vi "CLK6.vi"(11 "Queue Out":T1) -> (0 "error out":errorcluster)   [LabVIEW 2015]
uses:
  Class/Time.lvclass
  Global/SeverGlobal.vi
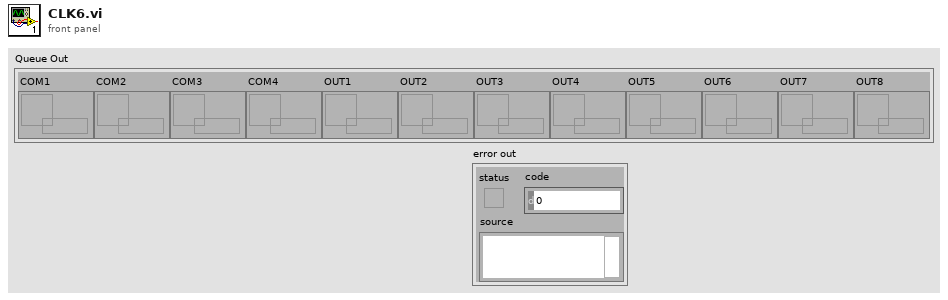
[diagram p1: front panel]
types:
  T1 = typedef "队列.ctl" = cluster{"COM1":refnum<queue>, "COM2":refnum<queue>, "COM3":refnum<queue>, "COM4":refnum<queue>, "OUT1":refnum<queue>, "OUT2":refnum<queue>, "OUT3":refnum<queue>, "OUT4":refnum<queue>, "OUT5":refnum<queue>, "OUT6":refnum<queue>, "OUT7":refnum<queue>, "OUT8":refnum<queue>}
  T2 = cluster{"TCP Ref":refnum<k5>, "IP":string, "userName":string, "A":u16, "COM":u16, "time":u32}
  T3 = cluster{"TCP Ref":refnum<k5>, "IP":string, "userName":string, "IN":u16, "OUT":u16, "time":u32}[]
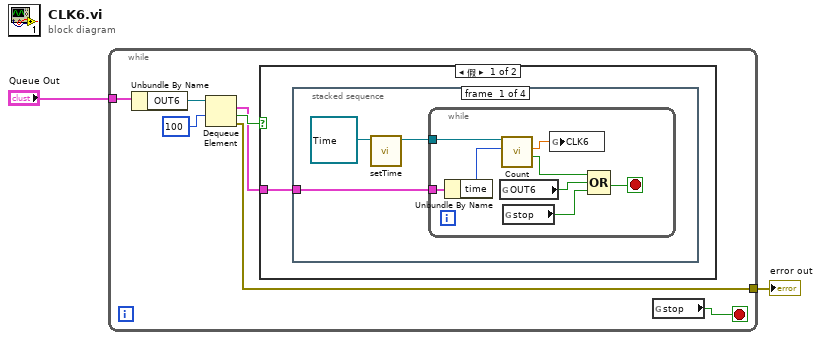
[diagram p0: block diagram]
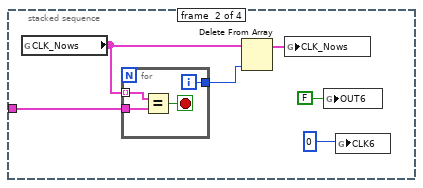
[diagram p2: hidden frame]
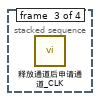
[diagram p3: hidden frame]
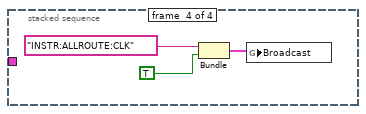
[diagram p4: hidden frame]
diagram:
  n1 = while {
    tunnel: "Queue Out" -> [w5]
    tunnel: [w3] -> w1
    stop <- w6 stop-if-true
    n2 = Unbundle By Name(w5) -> ("OUT6"=w4:refnum<queue>)
    n3 = Dequeue Element(queue=w4, timeout in ms (-1)=100) -> (element=w7:T2, timed out?=w8:bool, error out=w3:errorcluster)  [unwired: 1 in, 1 out]
    n4 = case shown="假" w8 {
      tunnel: w7 -> [w10 _]
      frame False {
        n5 = stacked-sequence {
          tunnel: w10 -> [w11 w26 _ _]
          frame #0 {
            n6 = call-dynamic "setTime.vi"("Time in"=refnum<class "Time.lvclass"> refnum ("Time.lvclass")) -> ("Time out"=w12:refnum<class "Time.lvclass">)  [unwired: 9 in, 1 out]
            n7 = while {
              tunnel: w12 -> [w21]
              tunnel: w11 -> [w20]
              stop <- w17 stop-if-true
              n8 = Unbundle By Name(w20) -> ("time"=w19:u32)
              n9 = global read "SeverGlobal.vi" "OUT6"() -> (w16:bool)
              n10 = call-dynamic "Count.vi"("计时"=w19, "Time in"=w21) -> ("Time has Elapsed"=w18:bool, "倒计时"=w15:dbl)  [unwired: 6 in, 2 out]
              n11 = global read "SeverGlobal.vi" "stop"() -> (w14:bool)
              n12 = global write "SeverGlobal.vi" "CLK6"(w15) -> ()
              n13 = Compound Arithmetic op=OR(w18, w16, w14) -> (w17:bool)
            }
          }
          frame #1 {
            n14 = global read "SeverGlobal.vi" "CLK_Nows"() -> (w25:T3)
            n15 = for {
              tunnel: w25 -> [w31] mode=indexing
              tunnel: w26 -> [w30]
              tunnel: [w28] -> w24
              i -> [w28]
              stop <- w29 stop-if-true
              n16 = Equal?(x=w31, y=w30) -> (x = y?=w29:bool)
            }
            n17 = Delete From Array(array=w25, index=w24) -> (array with subset deleted=w23:T3)  [unwired: 1 in, 1 out]
            n18 = global write "SeverGlobal.vi" "CLK_Nows"(w23) -> ()
            n19 = global write "SeverGlobal.vi" "OUT6"(FALSE ("COM1")) -> ()
            n20 = global write "SeverGlobal.vi" "CLK6"(0 ("COM1")) -> ()
          }
          frame #2 {
            n21 = call "释放通道后申请通道_CLK.vi"() -> ()  [unwired: 11 in, 1 out]
          }
          frame #3 {
            n22 = Bundle("format string"="INSTR:ALLROUTE:CLK", TRUE) -> (w34:cluster{"format string":string, bool})  [unwired: 1 in]
            n23 = global write "SeverGlobal.vi" "Broadcast"(w34) -> ()
          }
        }
      }
      frame True {
      }
    }
    n24 = global read "SeverGlobal.vi" "stop"() -> (w6:bool)
  }
  "error out" <- w1
